vi "VI Server_Get Menu Ring Item Names_SpreadSheetStringFormat.vi"(7 "Label":string, 8 "error in":errorcluster, 11 "VI Server Cluster":T1) -> (0 "error out":errorcluster, 1 "Control Reference":refnum<vi>, 3 "VI Server Cluster.DUP":T1, 4 "ItemNames.SpreadSheetFormat":string)   [LabVIEW 2020]
doc: "Returns item names (STR array) of the Menu Ring."
uses:
  VI Server_TypeDefs/VI Server_RefsCluster.ctl
  VI Server Toolkit LV2013.lvlib
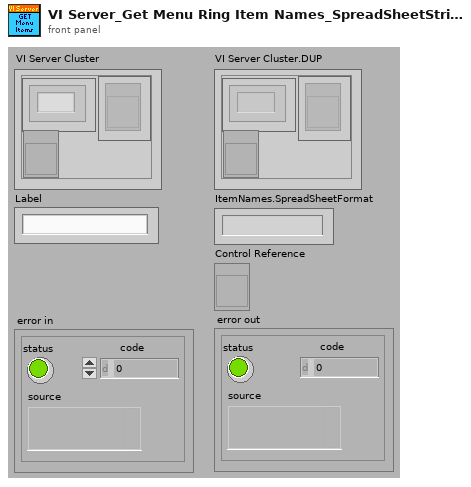
[diagram p1: front panel]
types:
  T1 = typedef "VI Server_RefsCluster.ctl" = cluster{"Labels":string[], "Refs":refnum<vi>[], "VI Ref":refnum<vi>}
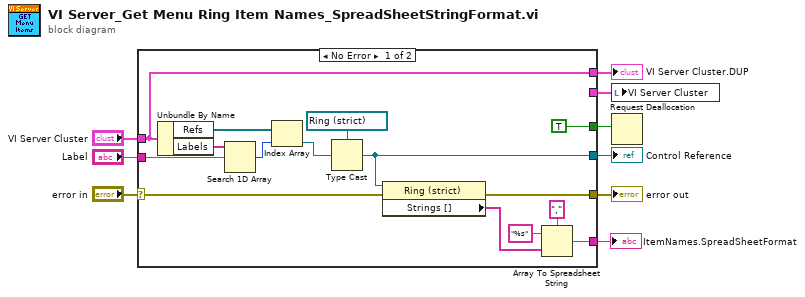
[diagram p0: block diagram]
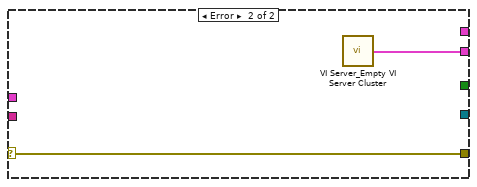
[diagram p2: hidden frame]
diagram:
  n1 = case shown="No Error" "error in" {
    selector: "error in" -> [w19 w26]
    tunnel: "Label" -> [w23 _]
    tunnel: "VI Server Cluster" -> [w16 _]
    tunnel: [w18 w26] -> w9
    tunnel: [w17 _] -> w5
    tunnel: [w16 _] -> w4
    tunnel: [TRUE _] -> w3
    tunnel: [_ w25] -> w2
    tunnel: [w10 _] -> w1
    frame No Error {
      n2 = Unbundle By Name(w16) -> ("Refs"=w21:refnum<vi>[], "Labels"=w24:string[])
      n3 = Search 1D Array(1D array=w24, element=w23) -> (index of element=w22:i32)  [unwired: 1 out]
      n4 = Index Array(array=w21, index=w22) -> (element=w20:refnum<vi>)
      n5 = Type Cast(type=refnum<vi> refnum ("Ring"), x=w20) -> (*(type *) &x=w17:refnum<vi>)
      n6 = property class="Ring (strict)"(reference=w17, error in=w19) -> (error out=w18:errorcluster, "Strings []"=w12:string[])  [unwired: 1 out]
      n7 = Array To Spreadsheet String(delimiter (Tab)=",", array=w12, 3:"%s" ("format string")) -> (spreadsheet string=w10:string)
    }
    frame Error {
      n8 = call "VI Server_Empty VI Server Cluster.vi"() -> ("VI Server Cluster"=w25:T1)  [unwired: 7 in]
    }
  }
  "error out" <- w9
  "VI Server Cluster.DUP" <- w4
  "Control Reference" <- w5
  "ItemNames.SpreadSheetFormat" <- w1
  n9 = local write "VI Server Cluster"(w2) -> ()
  n10 = Request Deallocation(w3) -> ()
